vi "SignalFilter.vi"(1 "Signal In":dbl) -> (0 "Filtered Signal":dynamicdata(graph))   [LabVIEW 2013]
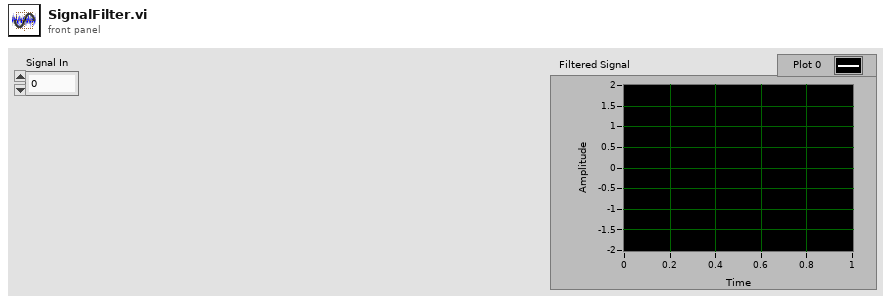
[diagram p1: front panel]
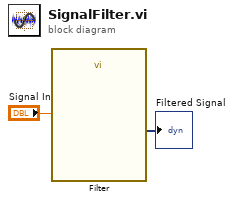
[diagram p0: block diagram]
diagram:
  n1 = call "Filter"("Signal"="Signal In") -> ("Filtered Signal"=→"Filtered Signal":dynamicdata)  [unwired: 9 in, 1 out]
